vi "10.1.-SubVI Decector de Renglones y Caracteres.vi"(8 "Boolean":bool, 10 "ARREGLO":i16[][](array[numeric]), 11 "INDICE":i32) -> (2 "FB":i32[](array[numeric]), 3 "FS":i32[](array[numeric]))   [LabVIEW 2020]
doc: "En este sub vi se guardan las posiciones del arreglo en donde se encuentran los flancos de subida y \nde bajada del arreglo. \n\nSe debe ingresar el arreglo a analizar y el indice para indicar si el análisis es para filas o columnas.\nfilas ---> 0 Y constante TRUE\ncolumas---->1 Y constante FALSE\n\n\n\nEl programa entrega dos arreglos en uno se encuentran los indices de los flancos de subida y en otros los de bajada."
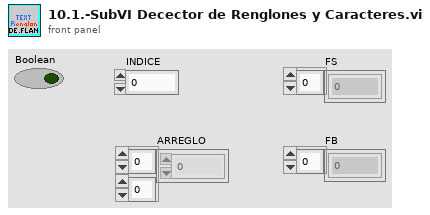
[diagram p1: front panel]
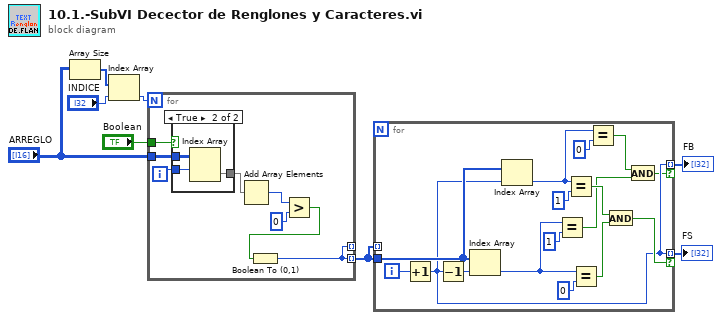
[diagram p0: block diagram]
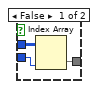
[diagram p2: hidden frame]
diagram:
  n1 = Array Size(array="ARREGLO") -> (size(s)=w5:i32[])
  n2 = Index Array "Index Array"(array=w5, index="INDICE") -> (element=w4:i32)
  n3 = for {
    N: w4 -> [_]
    tunnel: "ARREGLO" -> [w11]
    tunnel: [w13] -> w8 mode=indexing
    tunnel: [w13] -> _ mode=indexing
    tunnel: "Boolean" -> [w9]
    i -> [w12]
    n4 = case shown="True" w9 {
      tunnel: w11 -> [w19 w22]
      tunnel: [w18 w21] -> w10
      tunnel: w12 -> [w17 w20]
      frame False {
        n5 = Index Array(array=w19, index (col)=w17) -> (element=w18:i16[])  [unwired: 1 in]
      }
      frame True {
        n6 = Index Array(array=w22, index (row)=w20) -> (element=w21:i16[])  [unwired: 1 in]
      }
    }
    n7 = Add Array Elements(numeric array=w10) -> (sum=w16:i16)
    n8 = Greater?(x=w16, y=i16 0) -> (0:w14:bool)
    n9 = Boolean To (0,1)(Boolean=w14) -> (0, 1=w13:i16)
  }
  n10 = for {
    tunnel: w8 -> [w37]
    tunnel: [w24] -> w6 mode=indexing if=w25
    tunnel: [w24] -> w7 mode=indexing if=w23
    tunnel: w8 -> [_] mode=indexing
    i -> [w26]
    n11 = Increment(x=w26) -> (x+1=w24:i32)
    n12 = Decrement(x=w24) -> (x-1=w38:i32)
    n13 = Index Array "Index Array"(array=w37, index=w38) -> (element=w34:i16)
    n14 = Index Array "Index Array"(array=w37, index=w24) -> (element=w31:i16)
    n15 = Equal?(x=w34, y=i16 1) -> (x = y?=w27:bool)
    n16 = Equal?(x=w31, y=i16 1) -> (x = y?=w29:bool)
    n17 = Equal?(x=w34, y=i16 0) -> (x = y?=w30:bool)
    n18 = Equal?(x=w31, y=i16 0) -> (x = y?=w28:bool)
    n19 = And(x=w29, y=w30) -> (x .and. y?=w25:bool)
    n20 = And(x=w28, y=w27) -> (x .and. y?=w23:bool)
  }
  "FB" <- w7
  "FS" <- w6
